vi "Get Areas.vi"(5 "MetadataSize":u32, 6 "pMetadata":u32, 7 "DataSize":u32, 9 "pDataBuf":u32, 10 "timeout":u16, 11 "index":u16) -> (1 "pDataBuf out":u32, 3 "function return":i32, 4 "pMetadata out":u32)   [LabVIEW 2025, in "ExtremelyEpicImagerIPC2.lvlib"]
doc: "IMAGERIPC_API HRESULT WINAPI GetFrame2(WORD index, WORD timeout, void *pDataBuf, unsigned int DataSize, void *pMetadata, unsigned int MetadataSize); IMAGERIPC_API HRESULT WINAPI GetAreas(WORD index, WORD timeout, void *pDataBuf, unsigned int DataSize, void *pMetadata, unsigned int MetadataSize);"
uses:
  ExtremelyEpicImagerIPC2.lvlib
  ImagerIPC2.dll
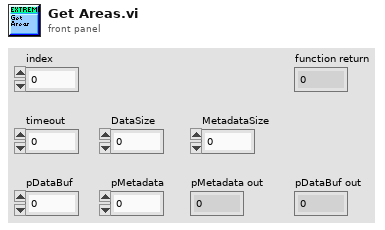
[diagram p1: front panel]
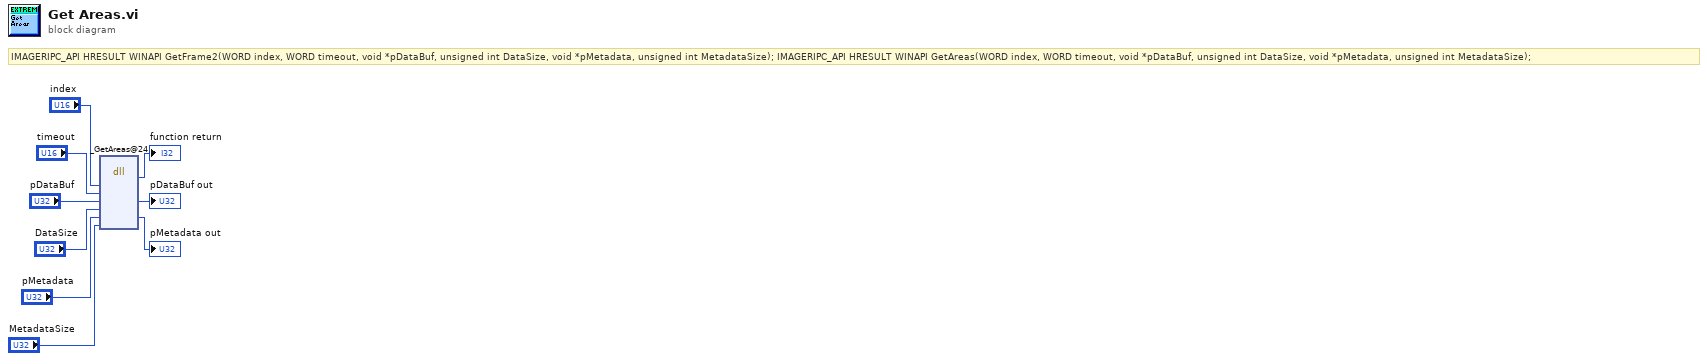
[diagram p0: block diagram]
diagram:
  # "IMAGERIPC_API HRESULT WINAPI GetFrame2(WORD index, WORD timeout, void *pDataBuf, unsigned int DataSize, void *pMetadata, unsigned int MetadataSize); IMAGERIPC_API HRESULT WINAPI GetAreas(WORD index, WORD timeout, void *pDataBuf, unsigned int DataSize, void *pMetadata, unsigned int MetadataSize);"
  n1 = dll-call lib="C:/Users/mayhe/OneDrive/Documents/GitHub/In-situ-monitoring-of-powder-bed-fusion-additive-manufacturing/system_development/Orichalcum/v0.2/Software_design/thermal-camera/VI/Connect SDK/ImagerIPC2.*" fn="_GetAreas@24"("index"="index", "timeout"="timeout", "pDataBuf"="pDataBuf", "DataSize"="DataSize", "pMetadata"="pMetadata", "MetadataSize"="MetadataSize") -> (→"function return":i32, "pDataBuf"=→"pDataBuf out":u32, "pMetadata"=→"pMetadata out":u32)  [unwired: 7 in, 2 out]
